vi "ConvertChannelQueryResponseToProperties.vi"(8 "error in (no error)":errorcluster, 11 "TektronixDPO_PhysicalDevice.lvclass":refnum<class "TektronixDPO_PhysicalDevice.lvclass">) -> (0 "error out":errorcluster, 3 "TektronixDPO_PhysicalDevice.lvclassOut":refnum<class "TektronixDPO_PhysicalDevice.lvclass">)   [LabVIEW 2013, in "TektronixDPO_PhysicalDevice.lvclass"]
doc: "Read from the phsyical device the offset relative to the specified channel"
uses:
  TektronixDPO_PhysicalDevice.lvclass
  shared/Typdefs/Choice78.ctl
  shared/Typdefs/Choice11.ctl
  shared/Typdefs/Choice79.ctl
  TektronixDPO_PhysicalDevice.lvclass/TektronixDPO_PhysicalDevice.ctl
panel:
  out "subarray":string[](array[string])
  # "Probe Gain"
  # "Bandwidth"
  # "Coupling"
  # "Offset"
  # "V/Division"
  # "Impedance"
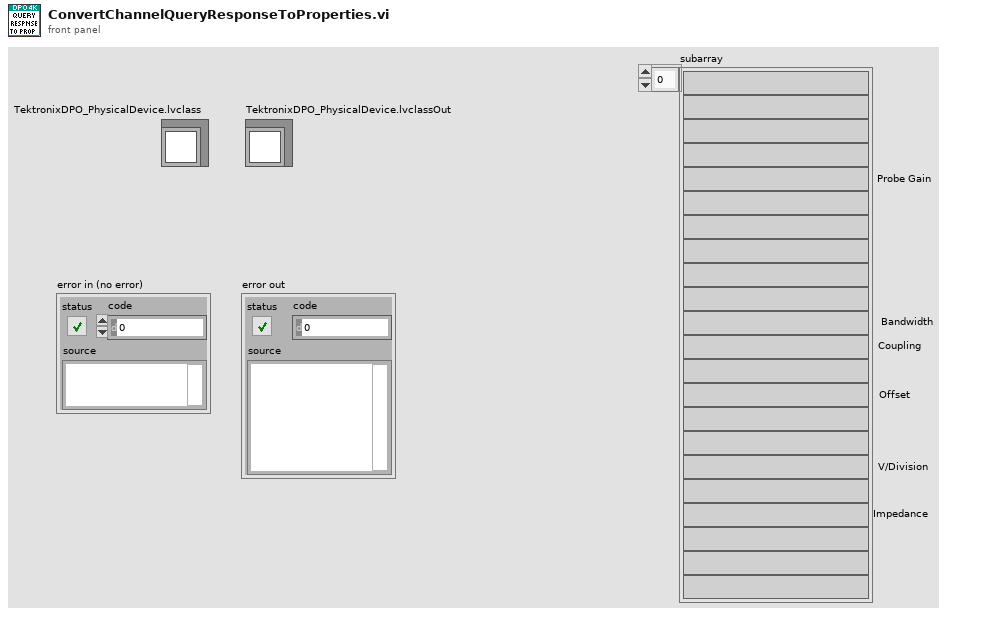
[diagram p1: front panel]
types:
  T1 = typedef "Choice79.ctl" = enum16{"FULL", "250 MHz", "150 MHz", "20 MHz"}
  T2 = typedef "Choice11.ctl" = enum16{"AC", "DC", "Ground"}
  T3 = typedef "Choice78.ctl" = enum16{"1M", "75", "50"}
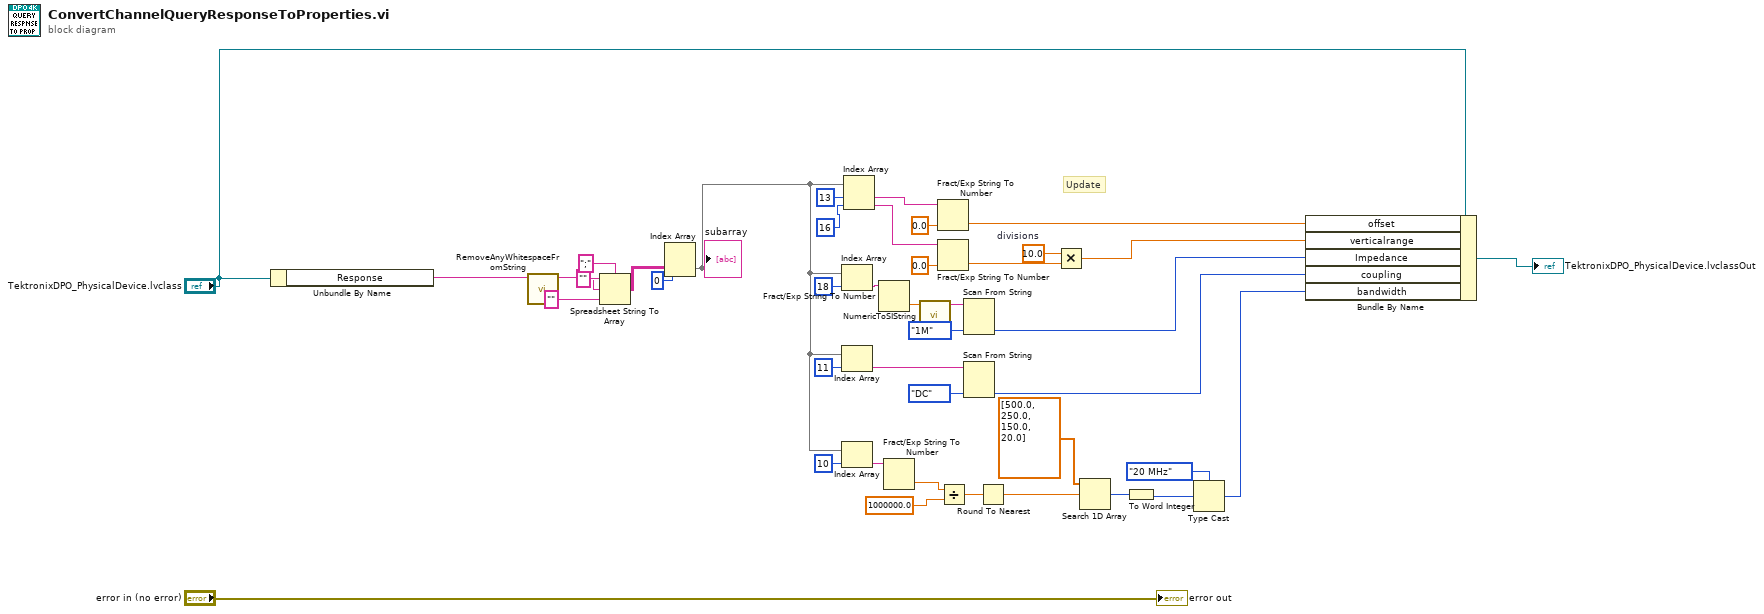
[diagram p0: block diagram]
diagram:
  w2 = 10.0  # divisions
  # "Update"
  n1 = Unbundle By Name("TektronixDPO_PhysicalDevice.lvclass") -> ("Response"=w32:string)
  n2 = call "RemoveAnyWhitespaceFromString.vi"("String in"=w32) -> ("String out"=w36:string)  [unwired: 10 in]
  n3 = Spreadsheet String To Array(delimiter (Tab)=";", format string="", spreadsheet string=w36, array type (2D Dbl)="") -> (array=w35:string[][])
  n4 = Index Array(array=w35, index (row)=0) -> (element=w33:string[])  [unwired: 1 in]
  "subarray" <- w33
  n5 = Index Array(array=w33, index=18) -> (element=w24:string)
  n6 = Index Array(array=w33, index=11) -> (element=w17:string)
  n7 = Index Array(array=w33, index=10) -> (element=w14:string)
  n8 = Index Array(array=w33, index #1=13 ("index"), index #2=16 ("index")) -> (element #1=w30:string, element #2=w26:string)
  n9 = Fract/Exp String To Number(string=w24) -> (number=w23:dbl)  [unwired: 3 in, 1 out]
  n10 = Fract/Exp String To Number(string=w14) -> (number=w13:dbl)  [unwired: 3 in, 1 out]
  n11 = call "NumericToSIString.vi"("Numeric"=w23) -> ("SI_String"=w22:string)  [unwired: 9 in, 1 out]
  n12 = Fract/Exp String To Number(string=w30, default (0 dbl)=0.0 ("default (0 DBL)")) -> (number=w31:dbl)  [unwired: 2 in, 1 out]
  n13 = Fract/Exp String To Number(string=w26, default (0 dbl)=0.0 ("default (0 DBL)")) -> (number=w27:dbl)  [unwired: 2 in, 1 out]
  n14 = Divide(x=w13, y=1000000.0) -> (x/y=w10:dbl)
  n15 = Scan From String(input string=w22, default 1=Choice78."1M" ("ActiveChannel.Impedance")) -> (output 1=w20:T3)  [unwired: 3 in, 3 out]
  n16 = Scan From String(input string=w17, default 1=Choice11."DC" ("Vertical Coupling (1: DC)")) -> (output 1=w16:T2)  [unwired: 3 in, 3 out]
  n17 = Round To Nearest(number=w10) -> (nearest integer value=w9:dbl)
  n18 = Multiply(x=w2, y=w27) -> (x*y=w3:dbl)
  n19 = Search 1D Array(1D array=dbl[] [500.0, 250.0, 150.0, 20.0], element=w9) -> (index of element=w8:i32)  [unwired: 1 in]
  n20 = To Word Integer(number=w8) -> (16bit integer=w6:i16)
  n21 = Type Cast(type=Choice79."20 MHz" ("Bandwidth"), x=w6) -> (*(type *) &x=w5:T1)
  n22 = Bundle By Name(cluster="TektronixDPO_PhysicalDevice.lvclass", "offset"=w31, "verticalrange"=w3, "Impedance"=w20, "coupling"=w16, "bandwidth"=w5) -> (→"TektronixDPO_PhysicalDevice.lvclassOut":refnum<class "TektronixDPO_PhysicalDevice.lvclass">)
  "error out" <- "error in (no error)"
